vi "Hex To Dec.vi"(1 "十六进制字符串":string) -> (7 "十进制整型字符串":string, 8 "十进制整数":i16, 9 "字符串":string)   [LabVIEW 2014]
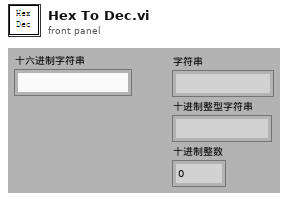
[diagram p1: front panel]
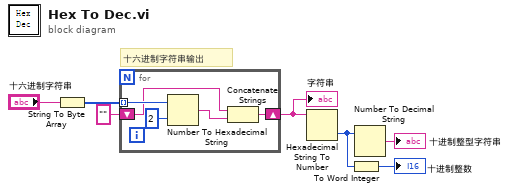
[diagram p0: block diagram]
diagram:
  # "十六进制字符串输出"
  n1 = String To Byte Array(string="十六进制字符串") -> (unsigned byte array=w7:u8[])
  n2 = for {
    tunnel: w7 -> [w12] mode=indexing
    shift-right: [w11] -> w5
    shift-left: "" -> [w10]
    n3 = Number To Hexadecimal String(1:i16 2 ("宽度(-)"), 2:w12) -> (0:w9:string)
    n4 = Concatenate Strings(w10, w9) -> (w11:string)
  }
  "字符串" <- w5
  n5 = Hexadecimal String To Number(string=w5) -> (number=w1:u32)  [unwired: 2 in, 1 out]
  n6 = To Word Integer(number=w1) -> (16bit integer=→"十进制整数":i16)
  n7 = Number To Decimal String(number=w1) -> (decimal integer string=→"十进制整型字符串":string)  [unwired: 1 in]
